vi "sample1.vi"() -> ()   [LabVIEW 2016]
uses:
  <vilib>/Math Plots/3D Math Plots/3D Surface/3D Surface XCtrl/3D Surface.xctl
  <vilib>/Math Plots/3D Math Plots/3D Surface/3D Surface Datatype/Public/Plot Helper (Vector).vi
  <vilib>/Math Plots/3D Math Plots/3D Surface/3D Surface Datatype/3D Surface Datatype.lvclass
panel:
  out "3D Surface":refnum<class "3D Plot Datatype.lvclass">[](xcontrol)
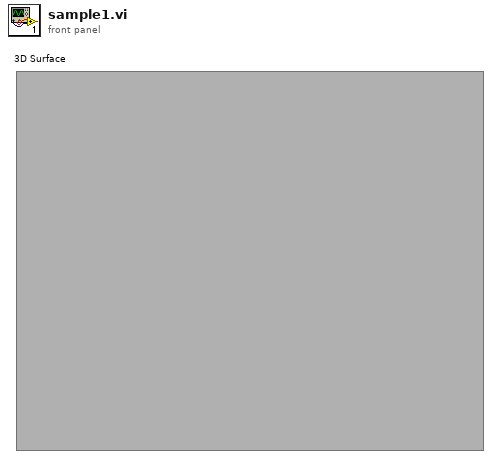
[diagram p1: front panel]
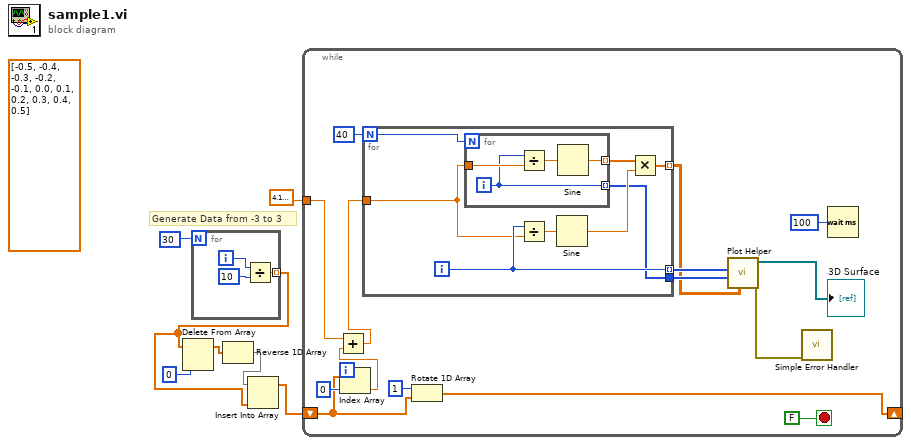
[diagram p0: block diagram]
diagram:
  (unwired) dbl[] [-0.5, -0.4, -0.3, -0.2, -0.1, 0.0, 0.1, 0.2, 0.3, 0.4, 0.5] ("Array")
  # "Generate Data from -3 to 3"
  n1 = for {
    N: 30 -> [_]
    tunnel: [w8] -> w1 mode=indexing
    i -> [w10]
    n2 = Divide(x=w10, y=10) -> (x/y=w8:dbl)
  }
  n3 = Delete From Array(array=w1, index=0) -> (array with subset deleted=w4:dbl[])  [unwired: 1 in, 1 out]
  n4 = Reverse 1D Array(array=w4) -> (reversed array=w3:dbl[])
  n5 = Insert Into Array(array=w3, new element=w1) -> (w2:dbl[])  [unwired: 1 in]
  n6 = while {
    shift-right: [w12] -> _
    shift-left: w2 -> [w13]
    tunnel: sgl 4.2 ("y") -> [w16]
    stop <- FALSE stop-if-true
    n7 = Index Array(array=w13, index=0) -> (element=w15:dbl)
    n8 = Add(x=w16, y=w15) -> (x+y=w14:dbl)
    n9 = for {
      N: 40 ("X input length") -> [w28]
      tunnel: [w30] -> w21 mode=indexing
      tunnel: [w29] -> w23 mode=indexing
      tunnel: [w27] -> w22
      tunnel: w14 -> [w26]
      i -> [w29]
      n10 = for {
        N: w28 -> [_]
        tunnel: [w36] -> w32 mode=indexing
        tunnel: w26 -> [w35]
        tunnel: [w34] -> w27 mode=indexing
        i -> [w34]
        n11 = Divide(x=w34, y=w35) -> (x/y=w37:dbl)
        n12 = Sine(x=w37) -> (sin(x)=w36:dbl)
      }
      n13 = Divide(x=w29, y=w26) -> (x/y=w33:dbl)
      n14 = Sine(x=w33) -> (sin(x)=w31:dbl)
      n15 = Multiply(x=w32, y=w31) -> (x*y=w30:dbl[])
    }
    n16 = Rotate 1D Array(1:w13, 2:1 ("n")) -> (0:w12:dbl[])
    n17 = call-poly <vilib>:"Plot Helper.vi"("z matrix"=w21, "y vector"=w22, "x vector"=w23) -> ("error out"=w19:errorcluster, "3D Plot lvclass Array out"=→"3D Surface":refnum<class "3D Plot Datatype.lvclass">[])  [unwired: 4 in, 3 out]
    n18 = call <vilib>:"Simple Error Handler.vi"("error in (no error)"=w19) -> ()  [unwired: 4 in, 5 out]
    n19 = Wait (ms)(milliseconds to wait=u32 100) -> ()  [unwired: 1 out]
  }
